vi "Robot Global Data.vi"() -> ()   [LabVIEW 2014]
doc: "This global VI can contain as many global variables as you need. Place a control on the panel, give it a good name. To read or write to it from a VI, drag the icon to the diagram of that VI. You can also drag from the project. Click on the node to change which global you access. You shouldn't have multiple locations writing to a global or it will cause a race-condition."
uses:
  <vilib>/Rock Robotics/WPI/Camera/WPI_CameraImageSize.ctl
  <vilib>/Rock Robotics/WPI/DriverStation/WPI_DriverStationRobotMode2.ctl
panel:
  out "Rate Motor A":dbl
  out "Distance A":dbl
  out "Lift Motor Settings":dbl[][][](array[numeric])=[[[0.25, -0.2], [0.38, -0.2]], [[0.48, -0.2], [0.5, -0.2]], [[0.55, 0.0], [0.57, 0.0]], [[0.7, -0.15], [0.6, -0.1]], [[0.6, -0.15], [0.7, -0.1]]]
  out "Rate Motor B":dbl
  out "HAT":i16
  out "Lift Motor A":dbl
  out "Distance B":dbl
  in  "Trigger":bool
  out "Lift Motor B":dbl
  in  "Arcade Drive?":bool
  in  "Robot Mode":T1
  in  "image size":T2=enum."320x240"
  in  "Enable Vision":bool
  # "Num"
  # "AB"
  # "Up Down"
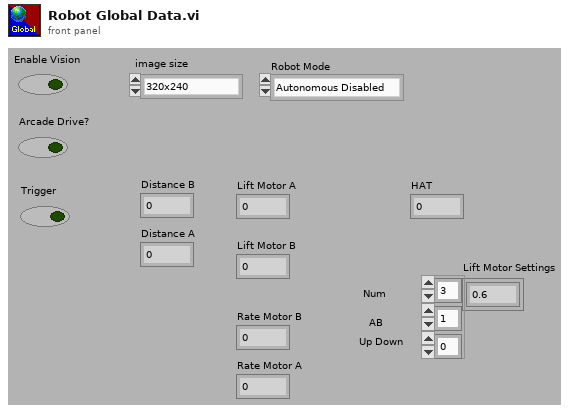
[diagram p1: front panel]
types:
  T1 = typedef "WPI_DriverStationRobotMode2.ctl" = enum16{"Autonomous Disabled", "Autonomous Enabled", "Teleop Disabled", "Teleop Enabled", "Disconnected", "Finish", "Test Disabled", "Test Enabled", "Emergency Stopped"}
  T2 = typedef "WPI_CameraImageSize.ctl" = enum16{"640x480", "320x240", "160x120", "Custom"}
diagram:
